vi "SendToServer.vi"() -> ()   [LabVIEW 2020]
uses:
  Subs/Server XCtrl/Server.xctl
  Subs/ColorText/Code.xctl
  Subs/Console XCtrl/Console_Xctrl.xctl
panel:
  out "Console_Xctrl":string(xcontrol)
  in  "Code":string(xcontrol)
  in  "Server":path(xcontrol)=path "/Users/crogers/GitHub/Summer2020/LabVIEWCode/Servers/Jens.vi"
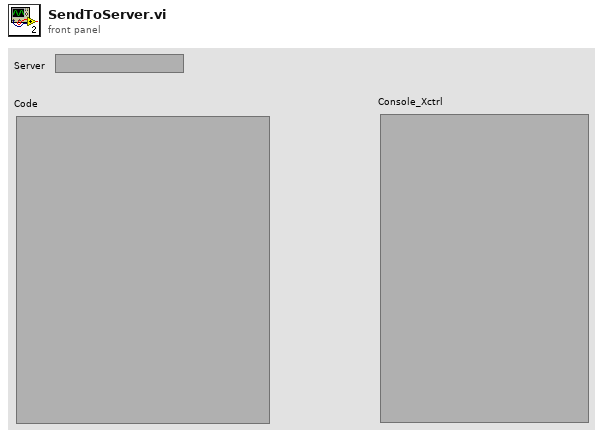
[diagram p1: front panel]
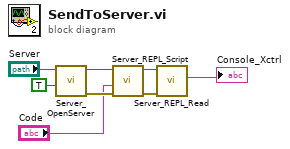
[diagram p0: block diagram]
diagram:
  n1 = call "Server_OpenServer.vi"("Wait for connection?"=TRUE, "Server"="Server") -> ("error out"=w5:errorcluster)  [unwired: 9 in]
  n2 = call "Server_REPL_Script.vi"("error in (no error)"=w5, "Code"="Code", "Server"="Server") -> ("error out"=w3:errorcluster)  [unwired: 8 in]
  n3 = call "Server_REPL_Read.vi"("error in (no error)"=w3, "Server"="Server") -> ("REPL"=→"Console_Xctrl":string)  [unwired: 7 in, 2 out]
